vi "Reconnect Count FG.vi"() -> (3 "s? t:f":i32)   [LabVIEW 2020, in "TCP Tests.lvlib"]
uses:
  TCP Tests.lvlib
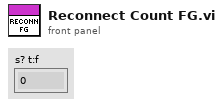
[diagram p1: front panel]
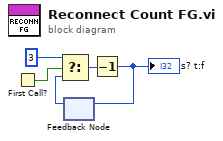
[diagram p0: block diagram]
diagram:
  n1 = First Call?() -> (First Call?: T/F=w5:bool)
  n2 = feedback #1() -> (w3:i32)  [unwired: 1 in]
  n3 = Select(t=3, s=w5, f=w3) -> (s? t:f=w2:i32)
  n4 = Decrement(x=w2) -> (x-1=w1:i32)
  "s? t:f" <- w1
  n5 = feedback-in #1(w1) -> ()
